vi "Example.vi"() -> ()   [LabVIEW 2015]
uses:
  Classes/slscsl/RelayPosition.ctl
  Classes/SLSC Switch/SLSC Switch.lvclass/SLSC Switch.ctl
  Classes/slscsl/RelayAction.ctl
  Classes/SLSC Switch/Connect Channels (Single).vi
  Classes/SLSC Switch/Connect Channels (Multiple).vi
  Classes/SLSC Switch/Disconnect Channels (Single).vi
  Classes/SLSC Switch/Disconnect Channels (Multiple).vi
  Classes/Relay Interface/RelayInterface.lvclass
  Classes/SLSC Switch/SLSC Switch.lvclass
  Classes/slscsl/slscsl.lvclass
panel:
  in  "Reload Topology":bool
  in  "Disconnect All":bool
  out "Active Connections":i32(listbox)
  in  "Tab Control":T1(tab)
  in  "Available Relays":i32[](listbox)
  in  "Open":bool
  in  "Close":bool
  in  "Channel A":i32(listbox)
  in  "Channel B":i32(listbox)
  in  "Disconnect":bool
  in  "Connect":bool
  in  "Add to List":bool
  in  "Connection List":string
  in  "Disconnect Multiple":bool
  in  "Connect Multiple":bool
  in  "Channel B":i32(listbox)
  in  "Channel A":i32(listbox)
  in  "Check Blacklist":bool
  in  "Channel A":i32(listbox)
  in  "Channel B":i32(listbox)
  in  "Remove from Blacklist":bool
  in  "Add to Blacklist":bool
  out "New Entry?":bool
  out "Found?":bool
  out "Relay Status":cluster{"RelayPosition":T2, "Name":string}[](array[cluster]) {"RelayPosition" items=["Open"=10, "Closed"=11]}
  out "error out":errorcluster
  in  "stop":bool
  in  "error in (no error)":errorcluster
  in  "Topology":string="BCI_VDT"
  in  "device":refnum<k21>="SLSC-12001-030EE1BD-Mod1"
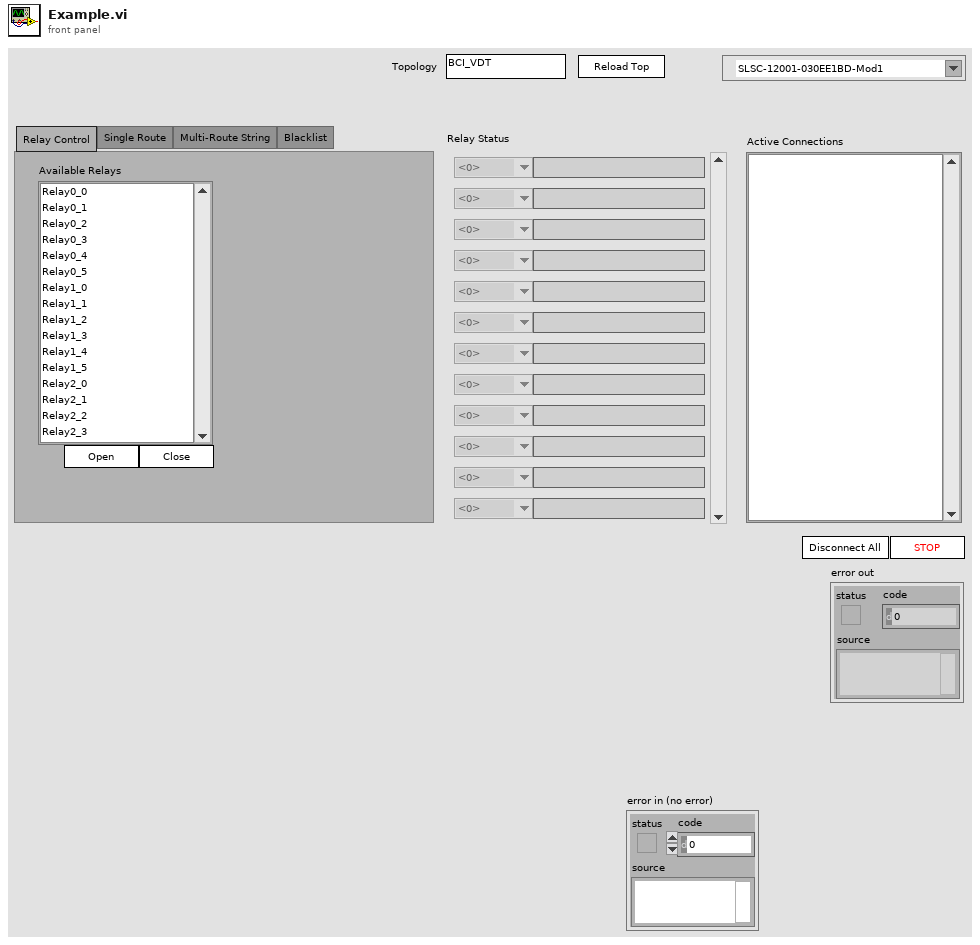
[diagram p1: front panel]
types:
  T1 = enum32{"Relay Control", "Single Route", "Multi-Route String", "Blacklist"}
  T2 = typedef "slscsl.lvclass/RelayPosition.ctl" = i32
  T3 = typedef "SLSC Switch.lvclass/Connection.ctl" = cluster{"channel 1":string, "channel 2":string}
  T4 = typedef "slscsl.lvclass/RelayAction.ctl" = u32
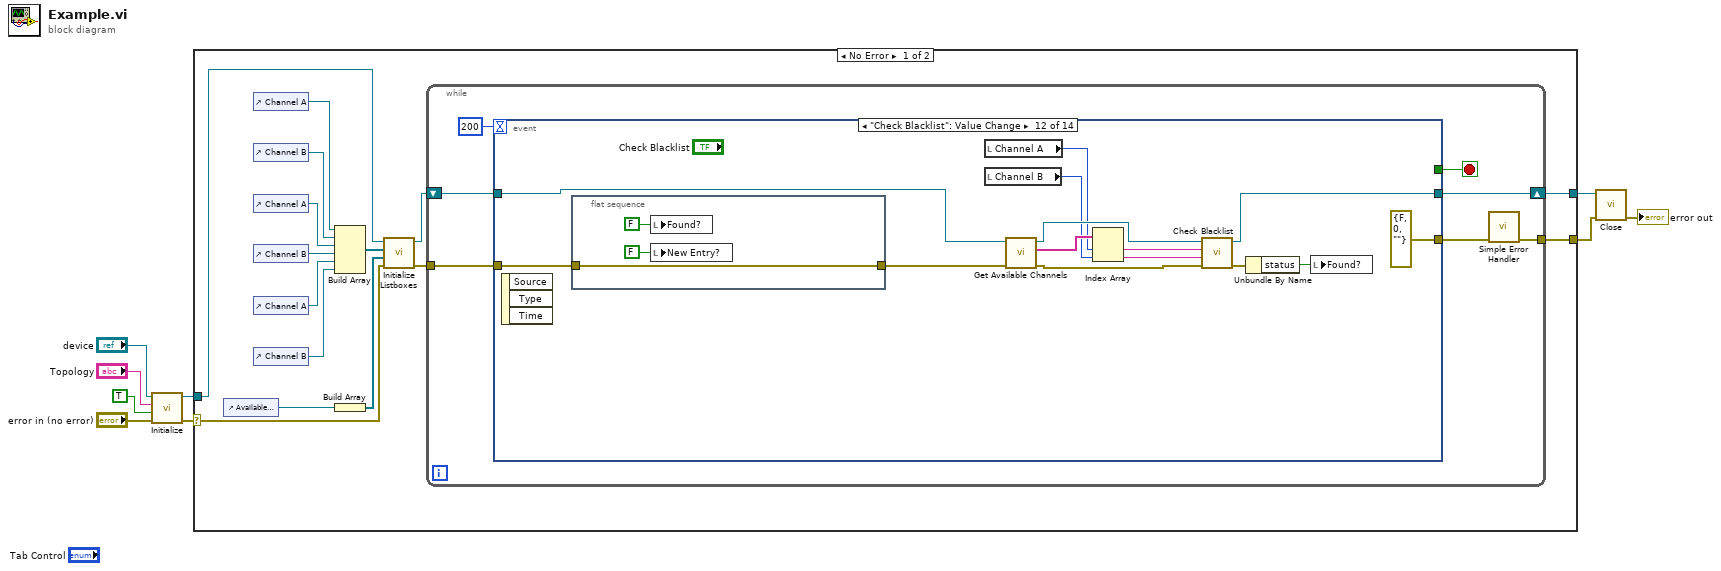
[diagram p0: block diagram]
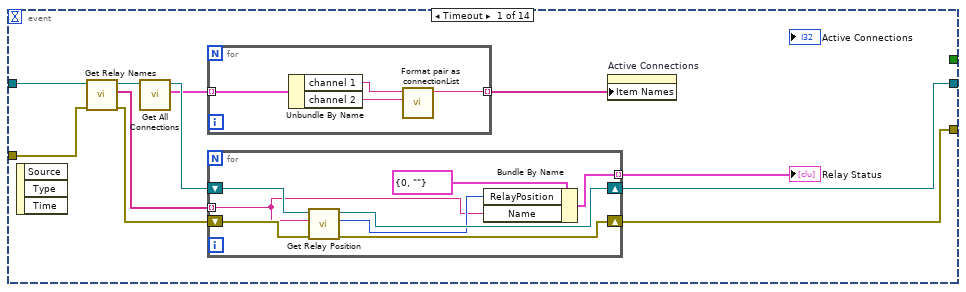
[diagram p2: hidden frame]
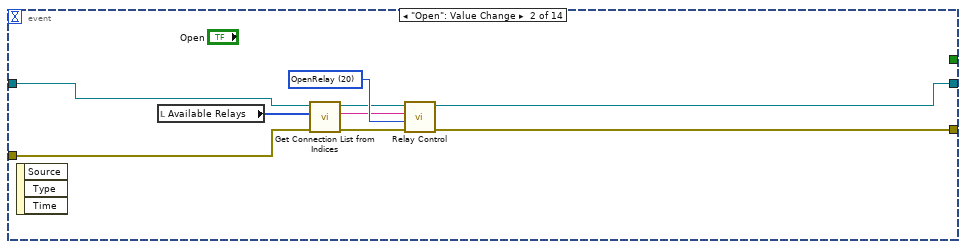
[diagram p3: hidden frame]
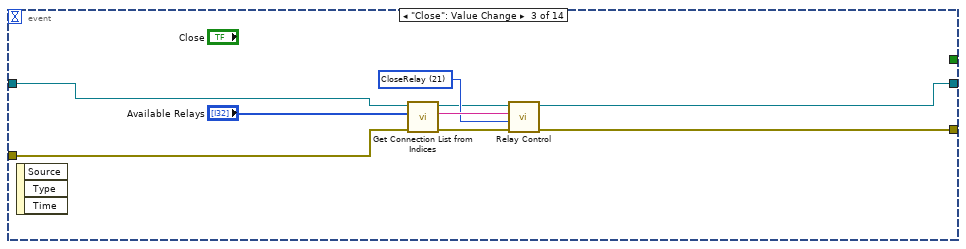
[diagram p4: hidden frame]
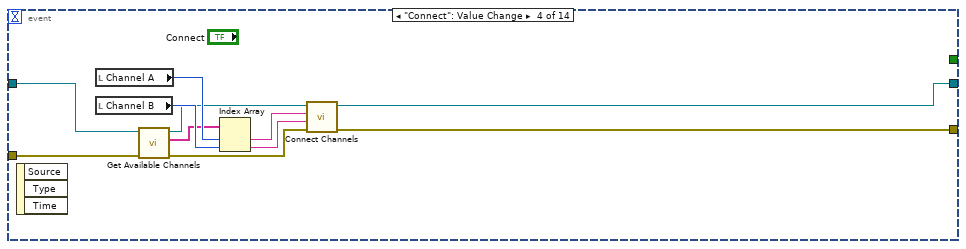
[diagram p5: hidden frame]
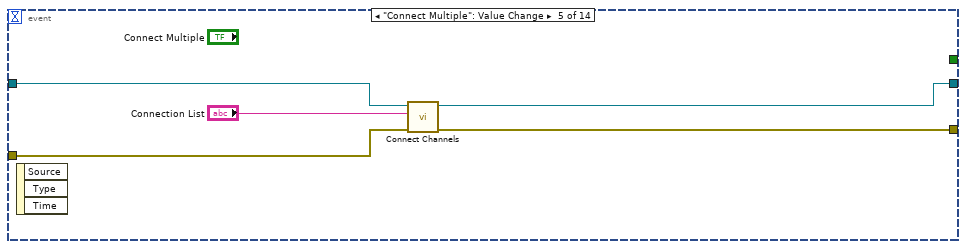
[diagram p6: hidden frame]
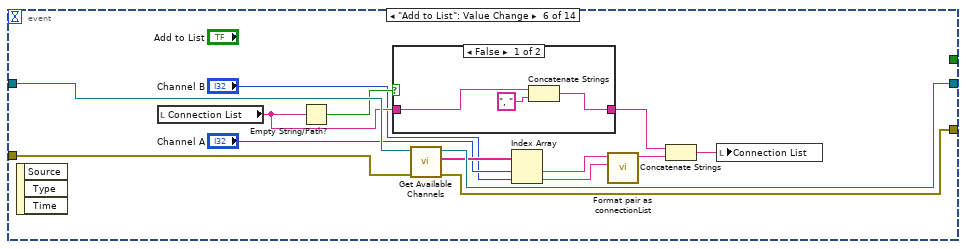
[diagram p7: hidden frame]
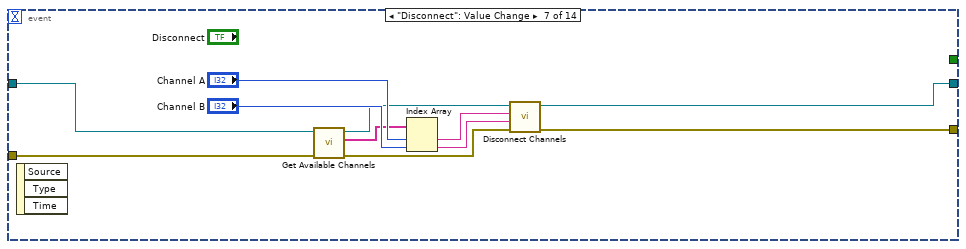
[diagram p9: hidden frame]
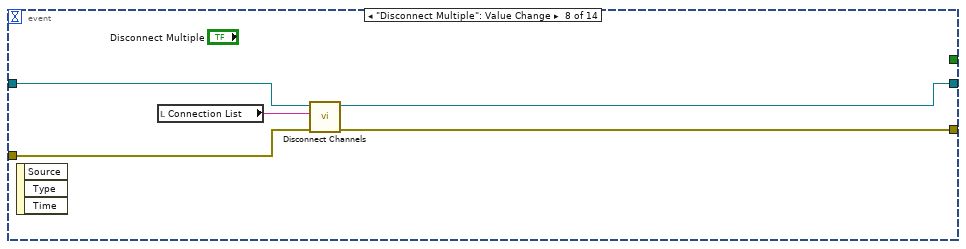
[diagram p10: hidden frame]
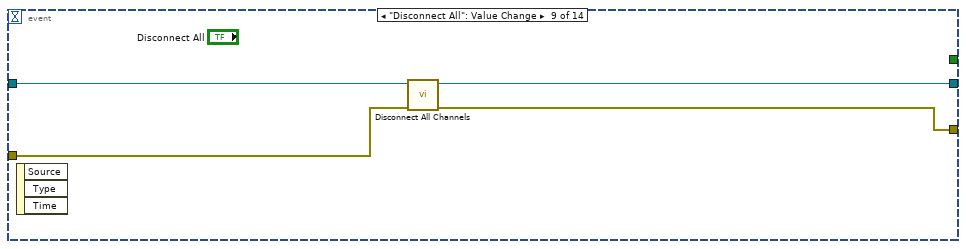
[diagram p11: hidden frame]
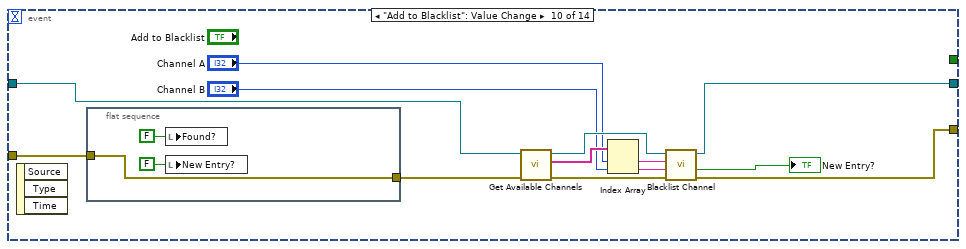
[diagram p12: hidden frame]
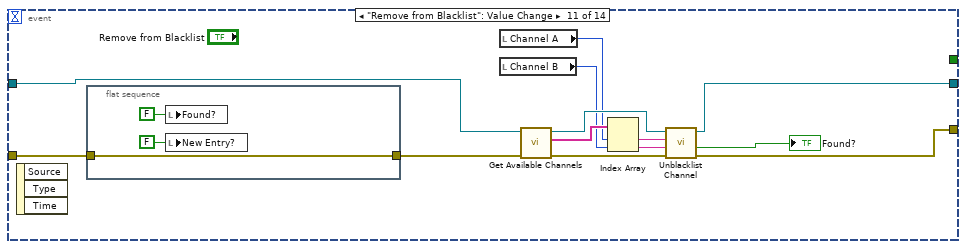
[diagram p13: hidden frame]
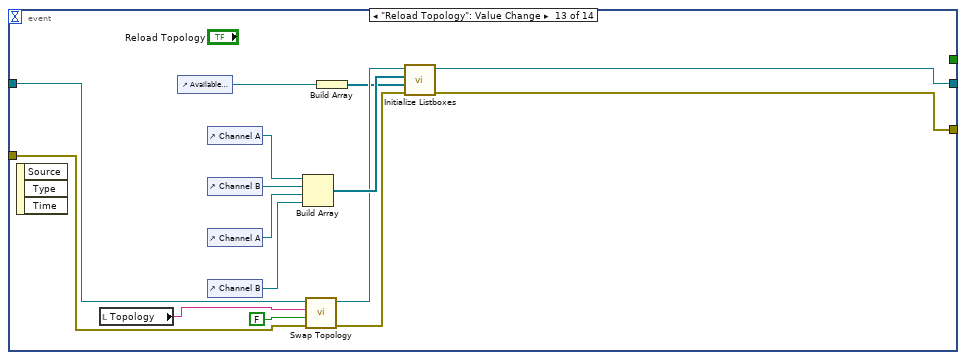
[diagram p14: hidden frame]
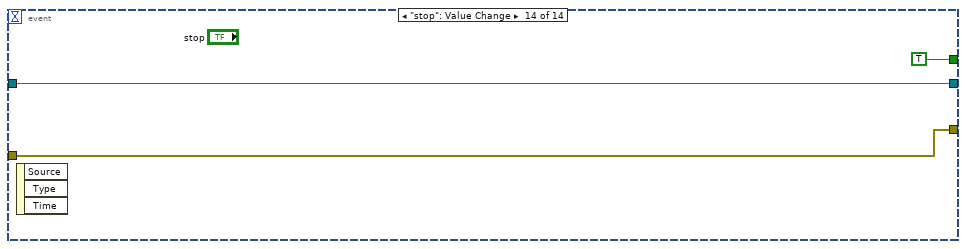
[diagram p15: hidden frame]
diagram:
  n1 = call "Initialize.vi"("error in (no error)"="error in (no error)", "reset device (boolean value)"=TRUE, "Topology"="Topology", "device"="device") -> ("error out"=w4:errorcluster, "SLSC Switch out"=w3:refnum<class "SLSC Switch.lvclass">)  [unwired: 6 in]
  n2 = case shown="No Error" w4 {
    selector: w4 -> [w14 w194]
    tunnel: [w24 w194] -> w7
    tunnel: [w23 w195] -> w6
    tunnel: w3 -> [w21 w195]
    frame No Error {
      n3 = control-ref of="Available Relays"() -> (w15:refnum<vi>)
      n4 = control-ref of="Channel A"() -> (w11:refnum<vi>)
      n5 = control-ref of="Channel B"() -> (w10:refnum<vi>)
      n6 = control-ref of="Channel A"() -> (w19:refnum<vi>)
      n7 = control-ref of="Channel B"() -> (w18:refnum<vi>)
      n8 = control-ref of="Channel A"() -> (w17:refnum<vi>)
      n9 = control-ref of="Channel B"() -> (w16:refnum<vi>)
      n10 = Build Array(w11, w10, w19, w18, w17, w16) -> (w13:refnum<vi>[])
      n11 = Build Array(w15) -> (w12:refnum<vi>[])
      n12 = call "Initialize Listboxes.vi"("error in (no error)"=w14, "Relay Boxes"=w12, "Channel Boxes"=w13, "SLSC Switch in"=w21) -> ("error out"=w20:errorcluster, "SLSC Switch out"=w22:refnum<class "SLSC Switch.lvclass">)  [unwired: 6 in]
      n13 = while {
        shift-right: [w29] -> w23
        shift-left: w22 -> [w30]
        tunnel: w20 -> [w31]
        tunnel: [w25] -> w24
        stop <- w27 stop-if-true
        n14 = event shown="[11] \"Check Blacklist\": Value Change" {
          selector: _ -> [_ _ _ _ _ _ _ _ _ _ _ _ _ _]
          dyn-events: _ -> [_ _ _ _ _ _ _ _ _ _ _ _ _ _]
          timeout: 200 -> [_ _ _ _ _ _ _ _ _ _ _ _ _ _]
          tunnel: w31 -> [w33 w56 w65 w74 w85 w101 w108 w120 w126 w136 w152 w172 w189 w193]
          tunnel: [w42 w63 w72 w82 w84 w99 w116 w119 w123 w138 w154 errorcluster {"status"=FALSE, "code"=0, "source"=""} ("error out") w177 w193] -> w26
          tunnel: w30 -> [w36 w60 w67 w77 w88 w102 w111 w122 w125 w135 w148 w170 w190 w192]
          tunnel: [w41 w62 w71 w83 w87 w100 w117 w121 w124 w139 w155 w164 w179 w192] -> w29
          tunnel: [_ _ _ _ _ _ _ _ _ _ _ _ _ TRUE] -> w27
          event Timeout {
            n15 = event-data() -> ()  [unwired: 1 in, 3 out]
            n16 = call "Get Relay Names.vi"("error in (no error)"=w33, "SLSC Switch in"=w36) -> ("error out"=w32:errorcluster, "Relay Names"=w34:string[], "SLSC Switch out"=w35:refnum<class "SLSC Switch.lvclass">)  [unwired: 7 in]
            n17 = call "Get All Connections.vi"("Route Manager in"=w35) -> ("connections"=w38:T3[], "Route Manager out"=w40:refnum<class "SLSC Switch.lvclass">)  [unwired: 9 in]
            n18 = for {
              tunnel: w38 -> [w46] mode=indexing
              tunnel: [w43] -> w37 mode=indexing
              n19 = Unbundle By Name(w46) -> ("channel 1"=w45:string, "channel 2"=w44:string)
              n20 = call "Format pair as connectionList.vi"("channel in"=w44, "channel 1"=w45) -> ("connectionList"=w43:string)  [unwired: 9 in]
            }
            n21 = for {
              shift-right: [w51] -> w41
              shift-left: w40 -> [w54]
              shift-right: [w52] -> w42
              shift-left: w32 -> [w53]
              tunnel: [w48] -> w39 mode=indexing
              tunnel: w34 -> [w47] mode=indexing
              n22 = call "Get Relay Position.vi"("error in (no error)"=w53, "relay name"=w47, "SLSC Switch in"=w54) -> ("error out"=w52:errorcluster, "position"=w49:T2, "SLSC Switch out"=w51:refnum<class "SLSC Switch.lvclass">)  [unwired: 6 in]
              n23 = Bundle By Name(cluster=cluster{"RelayPosition":T2, "Name":string} {"RelayPosition"=0, "Name"=""} ("Relay"), "RelayPosition"=w49, "Name"=w47) -> (w48:cluster{"RelayPosition":T2, "Name":string})
            }
            "Relay Status" <- w39
            n24 = property on="Active Connections" class="LstBox (strict)"("Item Names"=w37) -> ()  [unwired: 2 in, 2 out]
          }
          event "Open": Value Change {
            w61 = T4 20 items=["CloseRelay"=21, "OpenRelay"=20] ("RelayAction")
            n25 = event-data() -> ()  [unwired: 1 in, 3 out]
            n26 = local read "Available Relays"() -> (w57:i32[])
            n27 = call "Get Connection List from Indices.vi"("error in (no error)"=w56, "Available Relays"=w57, "SLSC Switch in"=w60) -> ("error out"=w55:errorcluster, "String"=w58:string, "SLSC Switch out"=w59:refnum<class "SLSC Switch.lvclass">)  [unwired: 6 in]
            n28 = call "Relay Control.vi"("error in (no error)"=w55, "relay action"=w61, "relay names"=w58, "SLSC Switch in"=w59) -> ("error out"=w63:errorcluster, "SLSC Switch out"=w62:refnum<class "SLSC Switch.lvclass">)  [unwired: 6 in]
          }
          event "Close": Value Change {
            w69 = T4 21 items=["CloseRelay"=21, "OpenRelay"=20] ("RelayAction")
            n29 = event-data() -> ()  [unwired: 1 in, 3 out]
            n30 = call "Get Connection List from Indices.vi"("error in (no error)"=w65, "Available Relays"="Available Relays", "SLSC Switch in"=w67) -> ("error out"=w64:errorcluster, "String"=w70:string, "SLSC Switch out"=w66:refnum<class "SLSC Switch.lvclass">)  [unwired: 6 in]
            n31 = call "Relay Control.vi"("error in (no error)"=w64, "relay action"=w69, "relay names"=w70, "SLSC Switch in"=w66) -> ("error out"=w72:errorcluster, "SLSC Switch out"=w71:refnum<class "SLSC Switch.lvclass">)  [unwired: 6 in]
          }
          event "Connect": Value Change {
            n32 = event-data() -> ()  [unwired: 1 in, 3 out]
            n33 = local read "Channel A"() -> (w79:i32)
            n34 = local read "Channel B"() -> (w78:i32)
            n35 = call "Get Available Channels.vi"("error in (no error)"=w74, "SLSC Switch in"=w77) -> ("error out"=w73:errorcluster, "Channels"=w75:string[], "SLSC Switch out"=w76:refnum<class "SLSC Switch.lvclass">)  [unwired: 7 in]
            n36 = Index Array(array=w75, index #1=w79, index #2=w78) -> (element #1=w81:string, element #2=w80:string)
            n37 = call-poly "Connect Channels.vi"("error in (no error)"=w73, "channel 2"=w80, "channel 1"=w81, "SLSC Switch in"=w76) -> ("error out"=w82:errorcluster, "SLSC Switch out"=w83:refnum<class "SLSC Switch.lvclass">)  [unwired: 6 in]
          }
          event "Connect Multiple": Value Change {
            n38 = event-data() -> ()  [unwired: 1 in, 3 out]
            n39 = call-poly "Connect Channels.vi"("error in (no error)"=w85, "connection list"="Connection List", "SLSC Switch in"=w88) -> ("error out"=w84:errorcluster, "SLSC Switch out"=w87:refnum<class "SLSC Switch.lvclass">)  [unwired: 7 in]
          }
          event "Add to List": Value Change {
            n40 = event-data() -> ()  [unwired: 1 in, 3 out]
            n41 = local read "Connection List"() -> (w96:string)
            n42 = Empty String/Path?(string/path=w96) -> (empty?=w97:bool)
            n43 = case shown="False" w97 {
              tunnel: w96 -> [w105 w106]
              tunnel: [w103 w106] -> w95
              frame False {
                n44 = Concatenate Strings(w105, ", " ("string")) -> (w103:string)
              }
              frame True {
              }
            }
            n45 = call "Get Available Channels.vi"("error in (no error)"=w101, "SLSC Switch in"=w102) -> ("error out"=w99:errorcluster, "Channels"=w98:string[], "SLSC Switch out"=w100:refnum<class "SLSC Switch.lvclass">)  [unwired: 7 in]
            n46 = Index Array(array=w98, index #1="Channel A", index #2="Channel B") -> (element #1=w94:string, element #2=w93:string)
            n47 = call "Format pair as connectionList.vi"("channel in"=w93, "channel 1"=w94) -> ("connectionList"=w92:string)  [unwired: 9 in]
            n48 = Concatenate Strings(w95, w92) -> (w91:string)
            n49 = local write "Connection List"(w91) -> ()
          }
          event "Disconnect": Value Change {
            n50 = event-data() -> ()  [unwired: 1 in, 3 out]
            n51 = call "Get Available Channels.vi"("error in (no error)"=w108, "SLSC Switch in"=w111) -> ("error out"=w107:errorcluster, "Channels"=w110:string[], "SLSC Switch out"=w109:refnum<class "SLSC Switch.lvclass">)  [unwired: 7 in]
            n52 = Index Array(array=w110, index #1="Channel A", index #2="Channel B") -> (element #1=w115:string, element #2=w114:string)
            n53 = call-poly "Disconnect Channels.vi"("error in (no error)"=w107, "channel 2"=w114, "channel 1"=w115, "SLSC Switch in"=w109) -> ("error out"=w116:errorcluster, "SLSC Switch out"=w117:refnum<class "SLSC Switch.lvclass">)  [unwired: 6 in]
          }
          event "Disconnect Multiple": Value Change {
            n54 = event-data() -> ()  [unwired: 1 in, 3 out]
            n55 = local read "Connection List"() -> (w118:string)
            n56 = call-poly "Disconnect Channels.vi"("error in (no error)"=w120, "disconnection list"=w118, "SLSC Switch in"=w122) -> ("error out"=w119:errorcluster, "SLSC Switch out"=w121:refnum<class "SLSC Switch.lvclass">)  [unwired: 7 in]
          }
          event "Disconnect All": Value Change {
            n57 = event-data() -> ()  [unwired: 1 in, 3 out]
            n58 = call "Disconnect All Channels.vi"("error in (no error)"=w126, "SLSC Switch in"=w125) -> ("error out"=w123:errorcluster, "SLSC Switch out"=w124:refnum<class "SLSC Switch.lvclass">)  [unwired: 8 in]
          }
          event "Add to Blacklist": Value Change {
            n59 = event-data() -> ()  [unwired: 1 in, 3 out]
            n60 = flat-sequence {
              tunnel: [w140] -> w133
              tunnel: w136 -> [w140]
              frame #0 {
                n61 = local write "Found?"(FALSE ("New Entry?")) -> ()
                n62 = local write "New Entry?"(FALSE ("New Entry?")) -> ()
              }
            }
            n63 = call "Get Available Channels.vi"("error in (no error)"=w133, "SLSC Switch in"=w135) -> ("error out"=w132:errorcluster, "Channels"=w131:string[], "SLSC Switch out"=w134:refnum<class "SLSC Switch.lvclass">)  [unwired: 7 in]
            n64 = Index Array(array=w131, index #1="Channel A", index #2="Channel B") -> (element #1=w128:string, element #2=w127:string)
            n65 = call "Blacklist Channel.vi"("error in (no error)"=w132, "Channel 2"=w127, "Channel 1"=w128, "SLSC Switch in"=w134) -> ("error out"=w138:errorcluster, "New Entry?"=→"New Entry?":bool, "SLSC Switch out"=w139:refnum<class "SLSC Switch.lvclass">)  [unwired: 5 in]
          }
          event "Remove from Blacklist": Value Change {
            n66 = event-data() -> ()  [unwired: 1 in, 3 out]
            n67 = flat-sequence {
              tunnel: [w156] -> w145
              tunnel: w152 -> [w156]
              frame #0 {
                n68 = local write "Found?"(FALSE ("New Entry?")) -> ()
                n69 = local write "New Entry?"(FALSE ("New Entry?")) -> ()
              }
            }
            n70 = local read "Channel A"() -> (w144:i32)
            n71 = local read "Channel B"() -> (w143:i32)
            n72 = call "Get Available Channels.vi"("error in (no error)"=w145, "SLSC Switch in"=w148) -> ("error out"=w146:errorcluster, "Channels"=w151:string[], "SLSC Switch out"=w147:refnum<class "SLSC Switch.lvclass">)  [unwired: 7 in]
            n73 = Index Array(array=w151, index #1=w144, index #2=w143) -> (element #1=w150:string, element #2=w149:string)
            n74 = call "Unblacklist Channel.vi"("error in (no error)"=w146, "Channel 2"=w149, "Channel 1"=w150, "SLSC Switch in"=w147) -> ("error out"=w154:errorcluster, "found?"=→"Found?":bool, "SLSC Switch out"=w155:refnum<class "SLSC Switch.lvclass">)  [unwired: 5 in]
          }
          event "Check Blacklist": Value Change {
            n75 = event-data() -> ()  [unwired: 1 in, 3 out]
            n76 = flat-sequence {
              tunnel: [w173] -> w167
              tunnel: w172 -> [w173]
              frame #0 {
                n77 = local write "Found?"(FALSE ("New Entry?")) -> ()
                n78 = local write "New Entry?"(FALSE ("New Entry?")) -> ()
              }
            }
            n79 = local read "Channel A"() -> (w166:i32)
            n80 = local read "Channel B"() -> (w165:i32)
            n81 = call "Get Available Channels.vi"("error in (no error)"=w167, "SLSC Switch in"=w170) -> ("error out"=w168:errorcluster, "Channels"=w171:string[], "SLSC Switch out"=w169:refnum<class "SLSC Switch.lvclass">)  [unwired: 7 in]
            n82 = Index Array(array=w171, index #1=w166, index #2=w165) -> (element #1=w163:string, element #2=w162:string)
            n83 = call "Check Blacklist.vi"("error in (no error)"=w168, "Channel 2"=w162, "Channel 1"=w163, "SLSC Switch in"=w169) -> ("error out"=w160:errorcluster, "SLSC Switch out"=w164:refnum<class "SLSC Switch.lvclass">)  [unwired: 5 in, 1 out]
            n84 = Unbundle By Name(w160) -> ("status"=w159:bool)
            n85 = local write "Found?"(w159) -> ()
          }
          event "Reload Topology": Value Change {
            n86 = event-data() -> ()  [unwired: 1 in, 3 out]
            n87 = local read "Topology"() -> (w187:string)
            n88 = control-ref of="Available Relays"() -> (w185:refnum<vi>)
            n89 = control-ref of="Channel A"() -> (w181:refnum<vi>)
            n90 = control-ref of="Channel B"() -> (w182:refnum<vi>)
            n91 = control-ref of="Channel A"() -> (w183:refnum<vi>)
            n92 = control-ref of="Channel B"() -> (w184:refnum<vi>)
            n93 = Build Array(w181, w182, w183, w184) -> (w186:refnum<vi>[])
            n94 = call "Swap Topology.vi"("error in (no error)"=w189, "reset device (boolean value)"=FALSE, "Topology"=w187, "SLSC Switch in"=w190) -> ("error out"=w178:errorcluster, "SLSC Switch out"=w180:refnum<class "SLSC Switch.lvclass">)  [unwired: 6 in]
            n95 = Build Array(w185) -> (w176:refnum<vi>[])
            n96 = call "Initialize Listboxes.vi"("error in (no error)"=w178, "Relay Boxes"=w176, "Channel Boxes"=w186, "SLSC Switch in"=w180) -> ("error out"=w177:errorcluster, "SLSC Switch out"=w179:refnum<class "SLSC Switch.lvclass">)  [unwired: 6 in]
          }
          event "stop": Value Change {
            n97 = event-data() -> ()  [unwired: 1 in, 3 out]
          }
        }
        n98 = call <vilib>:"Simple Error Handler.vi"("error in (no error)"=w26) -> ("error out"=w25:errorcluster)  [unwired: 4 in, 4 out]
      }
    }
    frame Error {
    }
  }
  n99 = call "Close.vi"("error in (no error)"=w7, "SLSC Switch in"=w6) -> ("error out"=→"error out":errorcluster)  [unwired: 9 in]
